vi "MenuConfig_LevelRead.vi"(8 "error in (no error)":errorcluster, 10 "Level.ID":string, 11 "MenuConfig":variant) -> (0 "error out":errorcluster, 2 "LevelConfig":T1, 3 "MenuConfig":variant)   [LabVIEW 2019, in "Menu Button.xctl"]
doc: "JSMA Module Template - Top Level UI 0.2.0.4\nRob Humfeld - Jet Engineering\nCopyright (c) 2019, Jet Engineering"
uses:
  Menu Button.xctl
  private/Level Config Cluster STYP.ctl
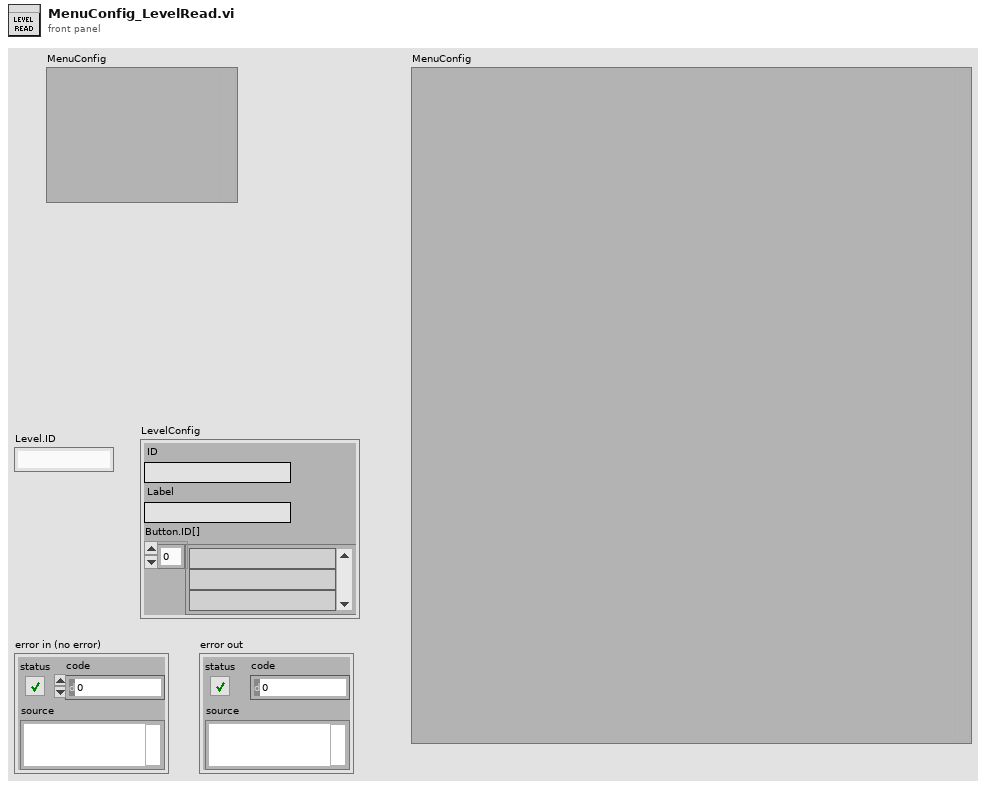
[diagram p1: front panel]
types:
  T1 = typedef "Menu Button.xctl/Level Config Cluster STYP.ctl" = cluster{"ID":string, "Label":string, "Button.ID[]":string[]}
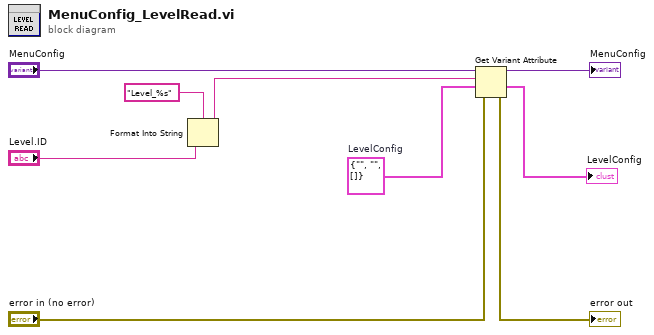
[diagram p0: block diagram]
diagram:
  w2 = T1 {"ID"="", "Label"="", "Button.ID[]"=[]}  # LevelConfig
  n1 = Format Into String(format string="Level_%s", "Level.ID") -> (resulting string=w3:string)  [unwired: 2 in, 1 out]
  n2 = Get Variant Attribute(Variant="MenuConfig", name=w3, default value (empty Variant)=w2, error in="error in (no error)") -> (duplicate Variant=→"MenuConfig":variant, value=→"LevelConfig":T1, error out=→"error out":errorcluster)  [unwired: 1 out]
